vi "Initialize Hardware.vi"(7 "hardware config file":path, 8 "error in":errorcluster, 10 "number of ports":i32, 11 "device parameters":T2) -> (0 "error out":errorcluster, 3 "hardware handles":T1)   [LabVIEW 2020, in "Ballard MIL-STD-1553 Engine.lvlib" / "Custom Device.lvlib"]
uses:
  Custom Device.lvlib
  Shared/Device Parameters.ctl
  Shared/Initialization Method.ctl
  <instrlib>/_AIM MIL-STD-1553/AIM Controls/1553 Select Direction.ctl
  AIM 1553 Examples/New Wrapped API/BC Transfer Descriptor.ctl
  Hardware Handles.ctl
panel:
  out "type string out":string
  out "product string out":string
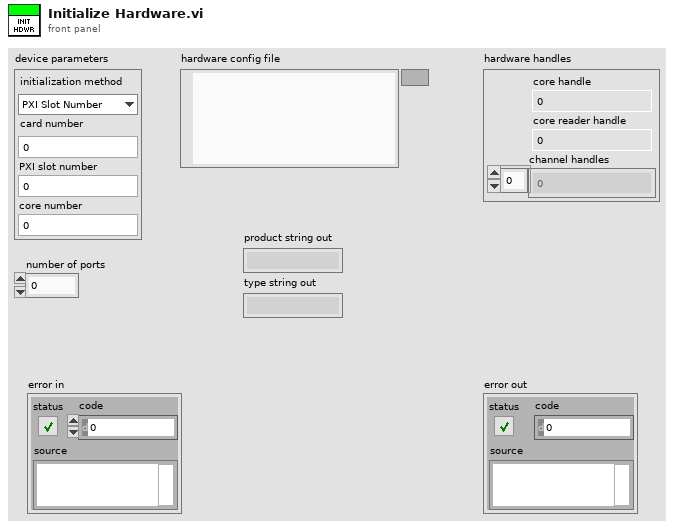
[diagram p1: front panel]
types:
  T1 = typedef "Ballard MIL-STD-1553 Engine.lvlib/Custom Device.lvlib/Hardware Handles.ctl" = cluster{"core handle":u64, "core reader handle":u64, "channel handles":u64[]}
  T2 = typedef "Device Parameters.ctl" = cluster{"initialization method":T3, "card number":i32, "PXI slot number":i32, "core number":i32}
  T3 = typedef "Initialization Method.ctl" = enum16{"PXI Slot Number", "Card Number"}
  T4 = cluster{"Transfer ID":u16, "BC Buffer Header ID":u16, "Transfer Type":enum16{"BC to RT transfer", "RT to BC transfer", "RT to RT transfer"}, "Receiving RT Address":u8, "Receiving RT Sub-address":u8}
  T5 = typedef "BC Transfer Descriptor.ctl" = cluster{"Transfer ID":u16, "Buffer Header ID":u16, "Transfer Type":enum16{"BC to RT transfer", "RT to BC transfer", "RT to RT transfer"}, "Bus":enum16{"primary", "secondary"}, "Transmitting RT Address":u8, "Receiving RT Address":u8, "Transmitting RT Sub-address":u8, "Receiving RT Sub-address":u8, "Word Count / Mode Code":u8, "Interrupt Control":enum16{"none", "on end of transfer", "on transfer error", "on status word exception"}, "Halt Control":enum16{"none", "on transfer error", "on status word exception", "on both", "on any interrupt"}, "Retry Control":enum16{"disable", "enable", "keep bus at next transmit", "alternate bus on next transmit"}, "Expected Response":enum16{"automatic", "no status word 1", "no status word 2"}, "Gap Mode":enum16{"delay", "standard", "fast"}, "Transfer Wait Time":u16}
  T6 = typedef "1553 Select Direction.ctl" = enum16{"receive", "transmit"}
  T7 = enum16{"BC to RT transfer", "RT to BC transfer", "RT to RT transfer"}
  T8 = typedef "Module Reference.ctl" = cluster{"Module Handle":u32, "BIU Number":u8}
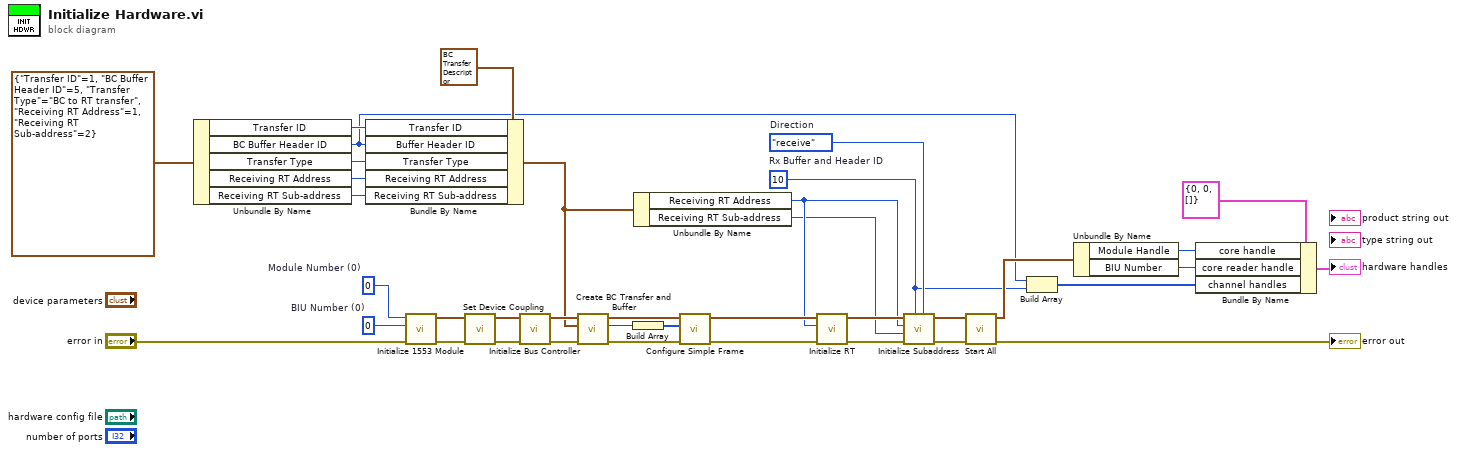
[diagram p0: block diagram]
diagram:
  w3 = u16 10  # Rx Buffer and Header ID
  w10 = 1553_Select_Direction."receive"  # Direction
  w20 = u8 0  # BIU Number (0)
  w21 = u32 0  # Module Number (0)
  n1 = Unbundle By Name(T4 {"Transfer ID"=1, "BC Buffer Header ID"=5, "Transfer Type"=enum."BC to RT transfer", "Receiving RT Address"=1, "Receiving RT Sub-address"=2} ("BC to RT Message Config")) -> ("Transfer ID"=w17:u16, "BC Buffer Header ID"=w4:u16, "Transfer Type"=w16:T7, "Receiving RT Address"=w15:u8, "Receiving RT Sub-address"=w14:u8)
  n2 = Bundle By Name(cluster=T5 {"Transfer ID"=1, "Buffer Header ID"=1, "Transfer Type"=enum."BC to RT transfer", "Bus"=enum."primary", "Transmitting RT Address"=0, "Receiving RT Address"=3, "Transmitting RT Sub-address"=0, "Receiving RT Sub-address"=13, "Word Count / Mode Code"=0, "Interrupt Control"=enum."none", "Halt Control"=enum."none", "Retry Control"=enum."disable", "Expected Response"=enum."automatic", "Gap Mode"=enum."delay", "Transfer Wait Time"=0} ("BC Transfer Descriptor"), "Transfer ID"=w17, "Buffer Header ID"=w4, "Transfer Type"=w16, "Receiving RT Address"=w15, "Receiving RT Sub-address"=w14) -> (w13:T5)
  n3 = call "Initialize 1553 Module.vi"("Error in"="error in", "BIU Number (0)"=w20, "Module Number (0)"=w21) -> ("Error out"=w37:errorcluster, "Module Reference out"=w33:T8)  [unwired: 7 in]
  n4 = call "Set Device Coupling.vi"("Error In (none)"=w37, "Module Reference"=w33) -> ("Error Out"=w38:errorcluster, "Module Reference out"=w32:T8)  [unwired: 8 in]
  n5 = call "Initialize Bus Controller.vi"("Error In"=w38, "Module Reference"=w32) -> ("Error Out"=w35:errorcluster, "Module Reference out"=w31:T8)  [unwired: 8 in]
  n6 = call "Create BC Transfer and Buffer.vi"("Error In"=w35, "BC Transfer Descriptor"=w13, "Module Reference"=w31) -> ("Error Out"=w34:errorcluster, "Transfer ID out"=w30:u16, "Module Reference out"=w29:T8)  [unwired: 6 in]
  n7 = Build Array(w30) -> (w36:u16[])
  n8 = Unbundle By Name(w13) -> ("Receiving RT Address"=w12:u8, "Receiving RT Sub-address"=w11:u8)
  n9 = call "Configure Simple Frame.vi"("Error In (none)"=w34, "Transfer IDs"=w36, "Module Reference"=w29) -> ("Error Out"=w28:errorcluster, "Module Reference out"=w23:T8)  [unwired: 7 in]
  n10 = call "Initialize RT.vi"("Error In"=w28, "RT Address"=w12, "Module Reference"=w23) -> ("Error Out"=w27:errorcluster, "Module Reference out"=w26:T8)  [unwired: 7 in]
  n11 = call "Initialize Subaddress.vi"("Direction (receive)"=w10, "Buffer Header and Buffer ID"=w3, "Error In"=w27, "Subaddress"=w11, "RT Address"=w12, "Module Reference"=w26) -> ("Error Out"=w25:errorcluster, "Module Reference out"=w24:T8)  [unwired: 4 in]
  n12 = call "Start All.vi"("Error In"=w25, "Module Reference"=w24) -> ("Error Out"=→"error out":errorcluster, "Module Reference out"=w7:T8)  [unwired: 8 in]
  n13 = Build Array(w4, w3) -> (w2:u16[])
  n14 = Unbundle By Name(w7) -> ("Module Handle"=w6:u32, "BIU Number"=w5:u8)
  n15 = Bundle By Name(cluster=T1 {"core handle"=0, "core reader handle"=0, "channel handles"=[]} ("hardware handles 2"), "core handle"=w6, "core reader handle"=w5, "channel handles"=w2) -> (→"hardware handles":T1)
